vi "HMI Connection.vi"(9 "Enum in":T1, 10 "reader endpoint":refnum<k21>, 11 "Refnum in":refnum<k21>) -> (1 "Enum out":T1)   [LabVIEW 2021]
uses:
  Controls/HMI-cRIO Connection Manager.ctl
  <resource>/objmgr/ni.dex.rc
panel:
  out "error out 2":errorcluster
  out "error out":errorcluster
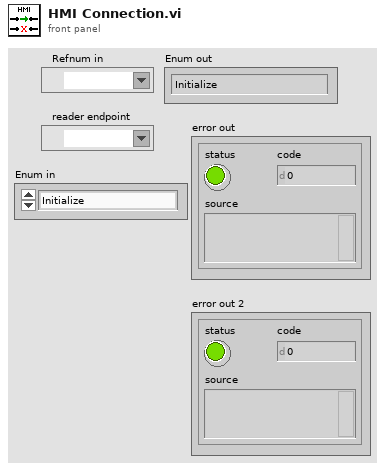
[diagram p1: front panel]
types:
  T1 = typedef "HMI-cRIO Connection Manager.ctl" = enum16{"Initialize", "Connect", "Connected"}
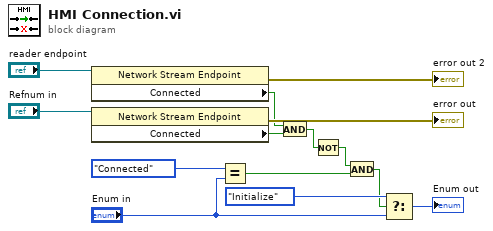
[diagram p0: block diagram]
diagram:
  n1 = property class="Network Stream Endpoint"(reference="reader endpoint") -> (error out=→"error out 2":errorcluster, "Connected"=w6:bool)  [unwired: 1 in, 1 out]
  n2 = property class="Network Stream Endpoint"(reference="Refnum in") -> (error out=→"error out":errorcluster, "Connected"=w5:bool)  [unwired: 1 in, 1 out]
  n3 = Equal?(x=HMI-cRIO_Connection_Manager."Connected", y="Enum in") -> (x = y?=w4:bool)
  n4 = And(x=w6, y=w5) -> (x .and. y?=w1:bool)
  n5 = Not(x=w1) -> (.not. x?=w2:bool)
  n6 = And(x=w2, y=w4) -> (x .and. y?=w3:bool)
  n7 = Select(t=HMI-cRIO_Connection_Manager."Initialize", s=w3, f="Enum in") -> (s? t:f=→"Enum out":T1)
